vi "CS POLARIS BME DG Client.unfold DIM Data.vi"(0 "Data":T1, 5 "error in (no error)":errorcluster) -> (13 "ErrorCode":i32, 14 "On":bool, 15 "output modulo":i32, 16 "RepRate":dbl, 17 "NextShot":dbl, 18 "DelayFormula":string="test", 19 "error out":errorcluster)   [LabVIEW 2009, in "CS POLARIS BME DG Client.lvlib"]
uses:
  CS POLARIS BME DG Client.lvlib
  CSCore/CSSystem/CoreDefs/CoreDefs.rawDataType.ctl
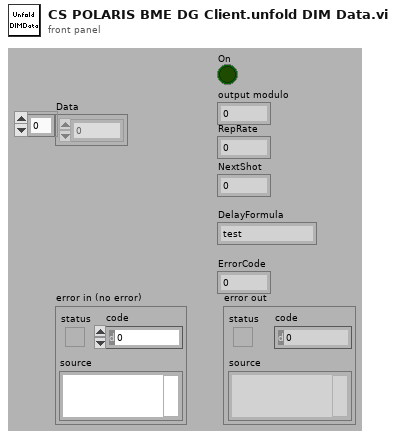
[diagram p1: front panel]
types:
  T1 = typedef "CoreDefs.rawDataType.ctl" = i8[]
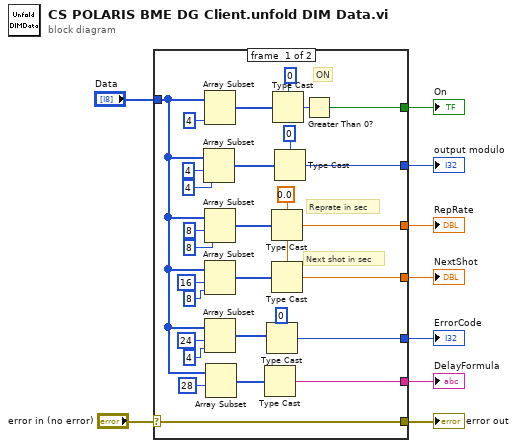
[diagram p0: block diagram]
diagram:
  n1 = case shown="No Error" "error in (no error)" {
    selector: "error in (no error)" -> [w20 w39]
    tunnel: [w20 w39] -> w8
    tunnel: "Data" -> [w23 _]
    tunnel: [w11 _] -> w1
    tunnel: [w19 _] -> w6
    tunnel: [w18 _] -> w5
    tunnel: [w17 _] -> w4
    tunnel: [w16 _] -> w3
    tunnel: [w15 _] -> w2
    frame #0 {
      w30 = 0.0 ("x")
      # "Next shot in sec"
      # "ON"
      # "Reprate in sec"
      n2 = Array Subset(array=w23, index=4, length=4) -> (w36:T1)
      n3 = Array Subset(array=w23, length=4 ("index")) -> (w10:T1)  [unwired: 1 in]
      n4 = Array Subset(array=w23, index=8, length=8) -> (w34:T1)
      n5 = Array Subset(array=w23, index=16, length=8) -> (w32:T1)
      n6 = Array Subset(array=w23, index=24, length=4) -> (w24:T1)
      n7 = Array Subset(array=w23, index=28) -> (w21:T1)  [unwired: 1 in]
      n8 = Type Cast(x=w21) -> (*(type *) &x=w19:string)  [unwired: 1 in]
      n9 = Type Cast(type=0 ("Numeric"), x=w24) -> (*(type *) &x=w18:i32)
      n10 = Type Cast(type=w30, x=w34) -> (*(type *) &x=w16:dbl)
      n11 = Type Cast(type=w30, x=w32) -> (*(type *) &x=w15:dbl)
      n12 = Type Cast(type=0 ("Numeric 2"), x=w10) -> (*(type *) &x=w13:i32)
      n13 = Type Cast(type=0 ("Numeric 2"), x=w36) -> (*(type *) &x=w17:i32)
      n14 = Greater Than 0?(x=w13) -> (x > 0?=w11:bool)
    }
    frame #1 {
    }
  }
  "error out" <- w8
  "output modulo" <- w4
  "DelayFormula" <- w6
  "ErrorCode" <- w5
  "RepRate" <- w3
  "NextShot" <- w2
  "On" <- w1
